vi "testCamera.vi"() -> ()   [LabVIEW 2009, in "run.lvlib"]
uses:
  run.lvlib
  Tools/Filing/FileSystem/FileSystem.lvclass
  Tools/CameraSettings/CamaraSettings.lvclass
  Channels/Camera/Camera/Camera.lvclass
  Tools/Filing/FileNeologist/FileNeologist.lvclass
panel:
  in  "number":i32=1
  out "stopped":bool
  out "imageSaved":bool
  out "temperature":dbl
  in  "stop":bool
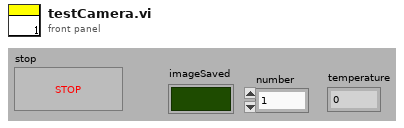
[diagram p1: front panel]
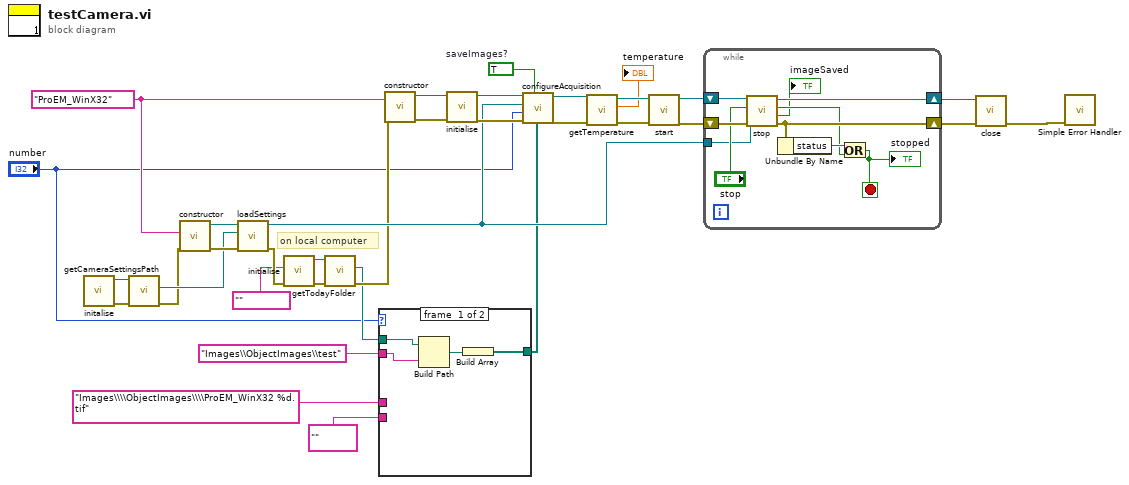
[diagram p0: block diagram]
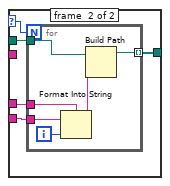
[diagram p2: hidden frame]
diagram:
  w12 = TRUE  # saveImages?
  w25 = "ProEM_WinX32" ("Camera")
  # "on local computer"
  n1 = call "initalise.vi"() -> ("error out"=w21:errorcluster, "FileSystem out"=w22:refnum<class "FileSystem.lvclass">)  [unwired: 10 in]
  n2 = call-dynamic "getCameraSettingsPath.vi"("error in (no error)"=w21, "FileSystem.lvclass in"=w22) -> ("error out"=w19:errorcluster, "CameraSettingsPath"=w20:path)  [unwired: 7 in, 1 out]
  n3 = call "constructor.vi"("error in (no error)"=w19, "camera settings"=w25) -> ("error out"=w23:errorcluster, "CamaraSettings out"=w24:refnum<class "CamaraSettings.lvclass">)  [unwired: 8 in]
  n4 = call-dynamic "loadSettings.vi"("error in (no error)"=w23, "Path"=w20, "CamaraSettings in"=w24) -> ("error out"=w17:errorcluster, "CamaraSettings out"=w18:refnum<class "CamaraSettings.lvclass">)  [unwired: 7 in]
  n5 = call "initialise.vi"("error in (no error)"=w17, "computer name"="") -> ("error out"=w15:errorcluster, "FileNeologist out"=w16:refnum<class "FileNeologist.lvclass">)  [unwired: 8 in]
  n6 = call "getTodayFolder.vi"("error in (no error)"=w15, "FileNeologist in"=w16) -> ("error out"=w9:errorcluster, "todayFolder"=w6:path)  [unwired: 7 in, 1 out]
  n7 = case shown="-1" "number" {
    selector: "number" -> [_ w40]
    tunnel: w6 -> [w37 w43]
    tunnel: [w38 w42] -> w1
    tunnel: "Images\\\\ObjectImages\\\\ProEM_WinX32 %d.tif" -> [_ w41]
    tunnel: "" -> [_ w39]
    tunnel: "Images\\ObjectImages\\test" -> [w36 _]
    frame #0 {
      n8 = Build Path(base path=w37, name or relative path=w36) -> (appended path=w35:path)
      n9 = Build Array(w35) -> (w38:path[])
    }
    frame #1 {
      n10 = for {
        N: w40 -> [_]
        tunnel: w43 -> [w49]
        tunnel: [w48] -> w42 mode=indexing
        tunnel: w41 -> [w46]
        tunnel: w39 -> [w44]
        i -> [w47]
        n11 = Format Into String(format string=w46, initial string=w44, w47) -> (resulting string=w45:string)  [unwired: 1 in, 1 out]
        n12 = Build Path(base path=w49, name or relative path=w45) -> (appended path=w48:path)
      }
    }
  }
  n13 = call "constructor.vi"("error in (no error)"=w9, "Camera"=w25) -> ("error out"=w26:errorcluster, "Camera out"=w34:refnum<class "Camera.lvclass">)  [unwired: 8 in]
  n14 = call-dynamic "initialise.vi"("error in (no error)"=w26, "Camera in"=w34) -> ("error out"=w27:errorcluster, "Camera out"=w33:refnum<class "Camera.lvclass">)  [unwired: 8 in]
  n15 = call-dynamic "configureAcquisition.vi"("imagePaths"=w1, "saveImages?"=w12, "error in (no error)"=w27, "number of Images"="number", "CameraSettings"=w18, "Camera in"=w33) -> ("error out"=w28:errorcluster, "Camera out"=w32:refnum<class "Camera.lvclass">)  [unwired: 4 in]
  n16 = call-dynamic "getTemperature.vi"("error in (no error)"=w28, "Camera in"=w32) -> ("error out"=w10:errorcluster, "temperature"=→"temperature":dbl, "Camera out"=w31:refnum<class "Camera.lvclass">)  [unwired: 7 in]
  n17 = call-dynamic "start.vi"("error in (no error)"=w10, "Camera in"=w31) -> ("error out"=w29:errorcluster, "Camera out"=w30:refnum<class "Camera.lvclass">)  [unwired: 8 in]
  n18 = while {
    tunnel: w18 -> [w55]
    shift-right: [w58] -> w11
    shift-left: w30 -> [w59]
    shift-right: [w54] -> w13
    shift-left: w29 -> [w57]
    stop <- w51 stop-if-true
    n19 = call-dynamic "stop.vi"("error in (no error)"=w57, "CameraSettings"=w55, "stop"="stop", "Camera in"=w59) -> ("error out"=w54:errorcluster, "imageSaved"=→"imageSaved":bool, "stopped?"=w52:bool, "Camera out"=w58:refnum<class "Camera.lvclass">)  [unwired: 4 in]
    n20 = Unbundle By Name(w54) -> ("status"=w53:bool)
    n21 = Or(x=w53, y=w52) -> (x .or. y?=w51:bool)
    "stopped" <- w51
  }
  n22 = call-dynamic "close.vi"("error in (no error)"=w13, "Camera in"=w11) -> ("error out"=w8:errorcluster)  [unwired: 9 in]
  n23 = call <vilib>:"Simple Error Handler.vi"("error in (no error)"=w8) -> ()  [unwired: 4 in, 5 out]
